vi "Parse Numeric.vi"(8 "error in (no error)":errorcluster, 10 "Index In":i32, 11 "JSON String":string) -> (0 "error out":errorcluster, 2 "Index Out":i32, 3 "JSON Value out":variant)   [LabVIEW 2017, in "JSON Support for LabVIEW.lvlib"]
uses:
  JSON Support for LabVIEW.lvlib
  Errors.ctl
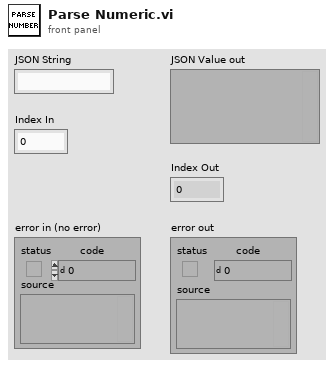
[diagram p1: front panel]
types:
  T1 = typedef "JSON Support for LabVIEW.lvlib/Errors.ctl" = enum16{"No key", "Key path type", "Array OOB", "Type Mismatch", "Invalid Token", "Invalid Value"}
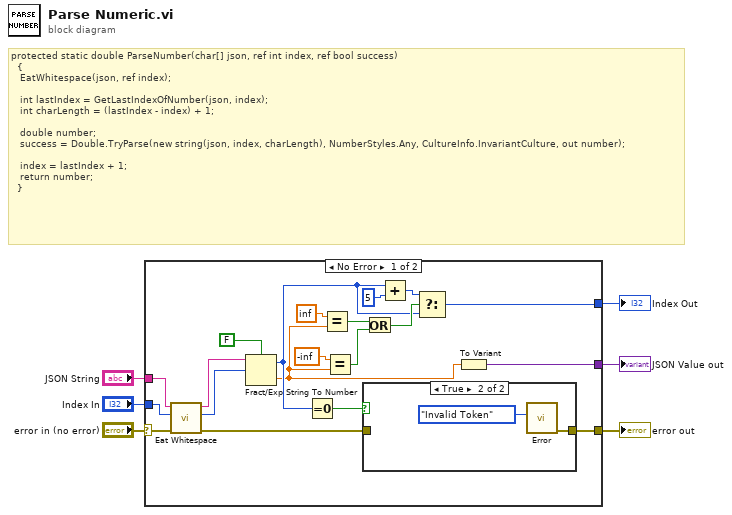
[diagram p0: block diagram]
diagram:
  # "protected static double ParseNumber(char[] json, ref int index, ref bool success)\n\t\t{\n\t\t\tEatWhitespace(json, ref index);\n\n\t\t\tint lastIndex = GetLastIndexOfNumber(json, index);\n\t\t\tint charLength = (lastIndex - index) + 1;\n\n\t\t\tdouble number;\n\t\t\tsuccess = Double.TryParse(new string(json, index, charLength), NumberStyles.Any, CultureInfo.InvariantCulture, out number);\n\n\t\t\tindex = lastIndex + 1;\n\t\t\treturn number;\n\t\t}"
  n1 = case shown="No Error" "error in (no error)" {
    selector: "error in (no error)" -> [w25 w30]
    tunnel: [w9 w30] -> w5
    tunnel: [w7 _] -> w1
    tunnel: "Index In" -> [w26 w31]
    tunnel: [w10 w31] -> w3
    tunnel: "JSON String" -> [w19 _]
    frame No Error {
      n2 = call "Eat Whitespace.vi"("error in (no error)"=w25, "Index In"=w26, "JSON String"=w19) -> ("error out"=w21:errorcluster, "Index Out"=w23:i32, "JSON String Passthrough"=w24:string)  [unwired: 6 in]
      n3 = Fract/Exp String To Number(use system decimal point (T)=FALSE, string=w24, offset=w23) -> (offset past number=w13:i32, number=w8:dbl)  [unwired: 1 in]
      n4 = Equal To 0?(x=w13) -> (x = 0?=w22:bool)
      n5 = Equal?(x=inf, y=w8) -> (x = y?=w17:bool)
      n6 = Equal?(x=-inf, y=w8) -> (x = y?=w15:bool)
      n7 = case shown="True" w22 {
        tunnel: w21 -> [w27 _]
        tunnel: [w27 w29] -> w9
        frame False {
        }
        frame True {
          n8 = call "Error.vi"(9:Errors."Invalid Token") -> ("error out"=w29:errorcluster)  [unwired: 9 in]
        }
      }
      n9 = Or(x=w17, y=w15) -> (x .or. y?=w14:bool)
      n10 = Add(x=w13, y=5) -> (x+y=w11:i32)
      n11 = Select(t=w11, s=w14, f=w13) -> (s? t:f=w10:i32)
      n12 = To Variant(anything=w8) -> (Variant=w7:variant)
    }
    frame Error {
    }
  }
  "error out" <- w5
  "Index Out" <- w3
  "JSON Value out" <- w1
